vi "about page.vi"   [LabVIEW 2016, in "FPGA Resource Manager System Defintion.lvlib"]
uses:
  FPGA Resource Manager System Defintion.lvlib
panel:
  # "NI Systems Engineering"
  # "FPGA Resource Manager"
  # "v1.0.0.1"
  # "https://github.com/LRUArchitecture/VeriStand-FPGA-Resource-Manager"
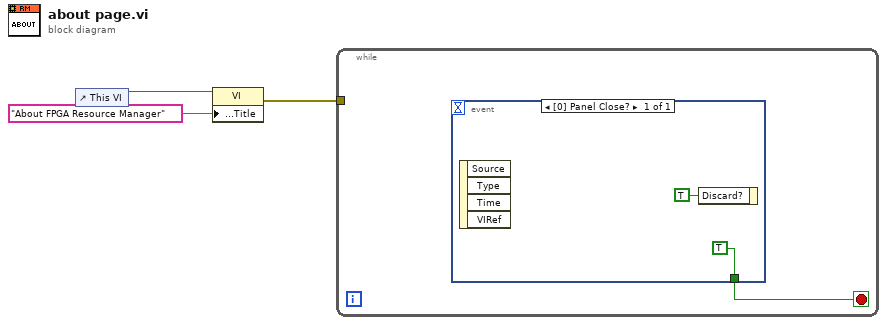
[diagram p0: block diagram]
diagram:
  n1 = control-ref of="This VI"() -> (w3:refnum<vi>)
  n2 = property class="VI"(reference=w3, "Front Panel.Title"="About FPGA Resource Manager" ("Front Panel Window:Title")) -> (error out=w1:errorcluster)  [unwired: 1 in, 1 out]
  n3 = while {
    tunnel: w1 -> [_]
    stop <- w4 stop-if-true
    n4 = event shown="[0] Panel Close?" {
      selector: _ -> [_]
      dyn-events: _ -> [_]
      timeout: _ -> [_]
      tunnel: [TRUE] -> w4
      event Panel Close? {
        n5 = event-data() -> ()  [unwired: 1 in, 4 out]
        n6 = event-data("Discard?"=TRUE) -> ()  [unwired: 1 in, 1 out]
      }
    }
  }
